vi "Rec New.vi"(4 "error in (no error)":errorcluster, 5 "mode (create new)":T1(ring), 6 "initial data":T2, 7 "object name (unnamed)":string) -> (0 "error out":errorcluster, 1 "status":enum16{"error", "new object", "existing object"}(ring), 3 "recordset reference":T4)   [LabVIEW 2013, in "NI_Database_API_64.lvlib"]
doc: "Looks up an existing <B>Recordset</B> object matching <B>object name</B> or creates a new Recordset object and returns a refnum you can use when calling other Recordset methods.\n\n<B>mode</B> specify whether you want to <B>create</B> a new object or <B>lookup</B> an existing object.\n\n<B>status</B> returns whether a new or an existing object reference is returned.\n\nObjects created with this VI should be destroyed using the <B>Rec Delete</B> VI."
uses:
  NI_Database_API_64.lvlib
  Rec ObjectReference.ctl
  Rec DataMembers.ctl
  Connection.llb/Conn ObjectReference.ctl
  <vilib>/Utility/_goopsup.llb/GOOP Object Repository Method.ctl
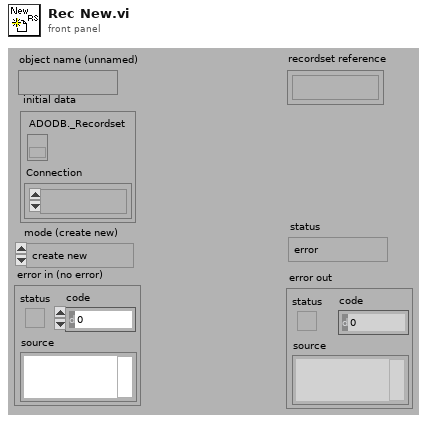
[diagram p1: front panel]
types:
  T1 = enum16{"create new", "lookup existing", "lookup or create"}
  T2 = typedef "NI_Database_API_64.lvlib/Rec DataMembers.ctl" = cluster{"ADODB._Recordset":refnum<k7>, "Connection":T3}
  T3 = typedef "NI_Database_API_64.lvlib/Conn ObjectReference.ctl" = refnum<k1>
  T4 = typedef "NI_Database_API_64.lvlib/Rec ObjectReference.ctl" = refnum<k1>
  T5 = typedef "GOOP Object Repository Method.ctl" = enum16{"Create", "GetCopy", "GetModify", "Set", "Destroy", "Create Static", "Get All Refs", "Reset", "Get Statistics"}
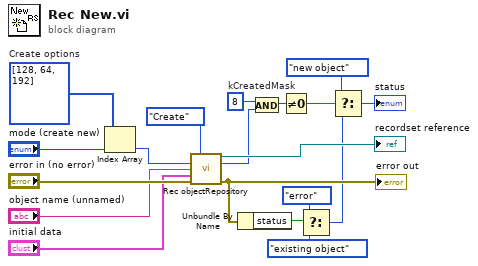
[diagram p0: block diagram]
diagram:
  w10 = i32[] [128, 64, 192]  # Create options
  w13 = 8  # kCreatedMask
  n1 = Index Array(array=w10, index="mode (create new)") -> (element=w9:i32)
  n2 = call "Rec objectRepository.vi"("method"=GOOP_Object_Repository_Method."Create", "flags in"=w9, "name in"="object name (unnamed)", "classDataIn"="initial data", "error in (no error)"="error in (no error)") -> ("recordset reference out"=→"recordset reference":T4, "flags out"=w12:i32, "error out"=w19:errorcluster)  [unwired: 4 in, 4 out]
  "error out" <- w19
  n3 = Unbundle By Name(w19) -> ("status"=w4:bool)
  n4 = And(x=w13, y=w12) -> (x .and. y?=w8:i32)
  n5 = Not Equal To 0?(x=w8) -> (x != 0?=w7:bool)
  n6 = Select(t=enum16{"error", "new object", "existing object"}."error" ("status"), s=w4, f=enum16{"error", "new object", "existing object"}."existing object" ("status")) -> (s? t:f=w2:enum16{"error", "new object", "existing object"})
  n7 = Select(t=enum16{"error", "new object", "existing object"}."new object" ("status"), s=w7, f=w2) -> (s? t:f=→"status":enum16{"error", "new object", "existing object"})
